vi "start.vi"(8 "error in (no error)":errorcluster, 11 "DistanceGauge in":refnum<class "DistanceGauge.lvclass">) -> (0 "error out":errorcluster, 3 "DistanceGauge out":refnum<class "DistanceGauge.lvclass">)   [LabVIEW 2013, in "DistanceGauge.lvlib" / "DistanceGauge.lvclass"]
uses:
  <userlib>/Common/Devices/DistanceGauge/DistanceGauge/DistanceGauge.lvclass
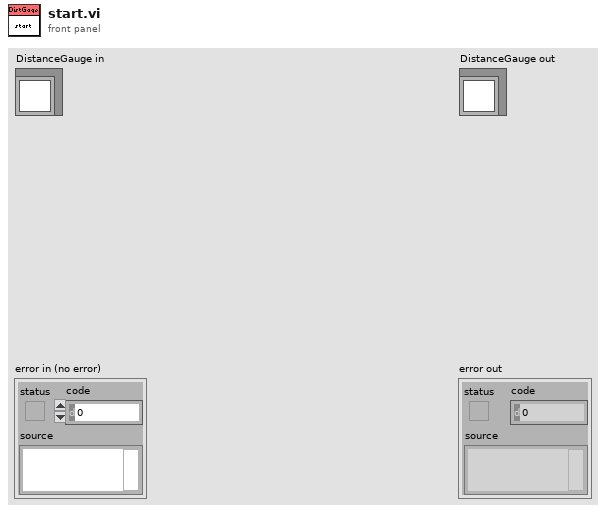
[diagram p1: front panel]
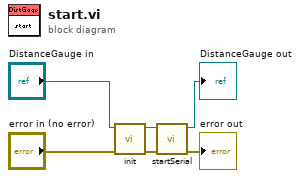
[diagram p0: block diagram]
diagram:
  n1 = call <userlib>:"init.vi"("error in (no error)"="error in (no error)", "DistanceGauge in"="DistanceGauge in") -> ("error out"=w1:errorcluster, "DistanceGauge out"=w3:refnum<class "DistanceGauge.lvclass">)  [unwired: 8 in]
  n2 = call <userlib>:"startSerial.vi"("error in (no error)"=w1, "DistanceGauge in"=w3) -> ("error out"=→"error out":errorcluster, "DistanceGauge out"=→"DistanceGauge out":refnum<class "DistanceGauge.lvclass">)  [unwired: 8 in]
